vi "ArdnoManualValvesFromUI.vi"(8 "error in (no error)":errorcluster, 10 "LINX Resource":T1, 11 "reference":refnum<vi>) -> (0 "error out":errorcluster)   [LabVIEW 2018, in "Arduino.lvlib"]
uses:
  Arduino.lvlib
  <vilib>/MakerHub/LINX/Private/Type Defs/LINX Ref.ctl
  <vilib>/MakerHub/LINX/Private/Type Defs/Platform.ctl
  <vilib>/MakerHub/LINX/Private/Type Defs/Interface.ctl
  <vilib>/MakerHub/LINX/Private/Device/Type Defs/LINX Device Config.ctl
  <vilib>/MakerHub/LINX/Private/Device/Type Defs/TCP Config.ctl
  <vilib>/MakerHub/LINX/Private/Device/Type Defs/Channels.ctl
  <vilib>/MakerHub/LINX/Public/Peripherals/Digital/Digital Write N Chans.vi
  <vilib>/MakerHub/LINX/Private/Local IO/LinxDigitalWrite.vi
  <vilib>/MakerHub/LINX/Public/Utilities/Check Channel.vi
  <vilib>/MakerHub/LINX/Private/Utilties/Generate Error.vi
  <vilib>/MakerHub/LINX/LMH-LINX.lvlib
  <vilib>/MakerHub/LINX/Private/Device/Device.lvlib
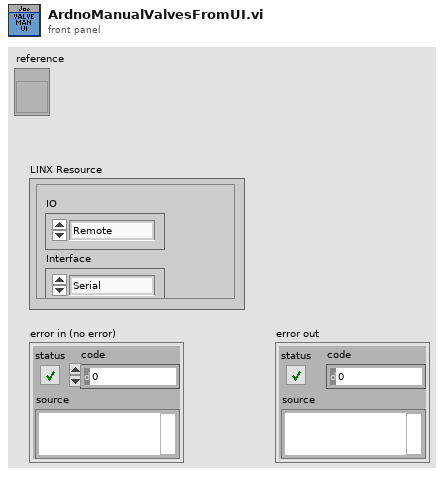
[diagram p1: front panel]
types:
  T1 = typedef "LMH-LINX.lvlib/LINX Ref.ctl" = cluster{"IO":T2, "Interface":T3, "LINX Device Config":T4}
  T2 = typedef "LMH-LINX.lvlib/Platform.ctl" = enum16{"Remote", "Local"}
  T3 = typedef "LMH-LINX.lvlib/Interface.ctl" = enum16{"Serial", "TCP"}
  T4 = typedef "LMH-LINX.lvlib/Device.lvlib/LINX Device Config.ctl" = cluster{"Interface":T3, "COM Port":refnum<visa-resource-name>, "TCP Configuration":T5, "Device Family":u8, "Device ID":u8, "Device Name":string, "TCP Ref":refnum<k5>, "Channels":T6}
  T5 = typedef "LMH-LINX.lvlib/Device.lvlib/TCP Config.ctl" = cluster{"IP Address":string, "Port":u16}
  T6 = typedef "LMH-LINX.lvlib/Channels.ctl" = cluster{"DI":u8[], "DO":u8[], "AI":u8[], "AO":u8[], "PWM":u8[], "QE":u8[], "UART":u8[], "I2C 2":u8[], "SPI":u8[], "CAN":u8[], "Servo":u8[], "AI Ref (V)":dbl, "AI Resolution (Bits)":u8, "AO Ref (V)":dbl, "AO Resolution (Bits)":u8}
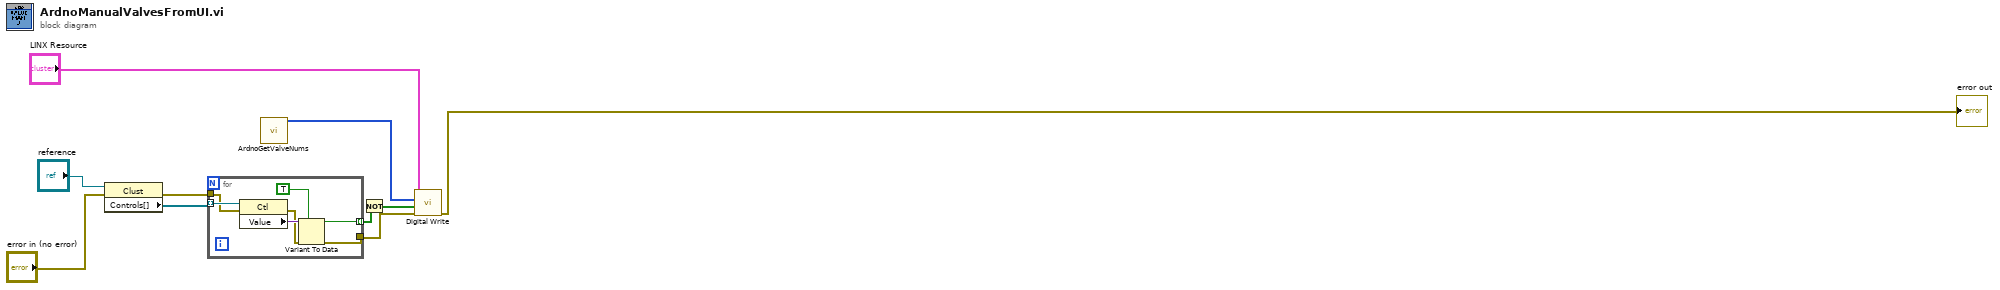
[diagram p0: block diagram]
diagram:
  n1 = property class="Clust"(reference="reference", error in="error in (no error)") -> (error out=w5:errorcluster, "Controls[]"=w4:refnum<vi>[])  [unwired: 1 out]
  n2 = for {
    tunnel: w4 -> [w17] mode=indexing
    tunnel: [w15] -> w9 mode=indexing
    tunnel: [w12] -> w8
    tunnel: w5 -> [w11]
    n3 = property class="Ctl"(reference=w17, error in=w11) -> (error out=w13:errorcluster, "Value"=w16:variant)  [unwired: 1 out]
    n4 = Variant To Data(error in=w13, type=TRUE, Variant=w16) -> (data=w15:bool, error out=w12:errorcluster)
  }
  n5 = call "ArdnoGetValveNums.vi"() -> ("Array"=w2:i32[])  [unwired: 11 in]
  n6 = Not(x=w9) -> (.not. x?=w1:bool[])
  n7 = call-poly <vilib>:"Digital Write.vi"("Error In"=w8, "Values"=w1, "DO Channels"=w2, "LINX Resource"="LINX Resource") -> ("Error Out"=→"error out":errorcluster)  [unwired: 6 in, 1 out]
